vi "Constants.vi"() -> ()   [LabVIEW 2020, in "Ballard MIL-STD-1553 Scripting.lvlib"]
doc: "Use this Global VI to access the GUIDs assigned to the page resources of the Custom Device."
uses:
  Ballard MIL-STD-1553 Scripting.lvlib
panel:
  in  "Tab Control":enum32{"GUIDs", "Constants", "Properties"}(tab)
  in  "GUID.Error Count Channel":string="28D1D890-3AED-4F6D-A978-AD9A95C11628"
  in  "GUID.Status Section":string="1E0B5C0B-62AA-4583-9D0D-4E49A372EA3D"
  in  "GUID.Command Channel":string="F3C769CE-2055-47DC-98AC-89CDFED404B4"
  in  "GUID.Acyclic Frames":string="E577908A-4C92-429B-8C68-9740E425B266"
  in  "GUID.Timestamp Channel":string="4F0EA705-FD0A-4F01-AD6C-880781D6ED5B"
  in  "GUID.Status Word":string="7948DA20-805D-45D0-914D-274A69BA1942"
  in  "GUID.Trigger Channel":string="9F1749FA-E57B-4A2B-A4F8-443BB28943E1"
  in  "GUID.Message":string="2151C088-5813-42CA-818D-390AC9DDD1E2"
  in  "GUID.Subaddress":string="7E2EB233-E0C6-4644-BE22-C64B35DA4442"
  in  "GUID.Remote Terminal":string="D816BAC3-B801-4086-8FF2-44DEB0EE8E0A"
  in  "GUID.Bus Controller":string="B770364E-A524-47A4-BD2C-84D1536BF350"
  in  "GUID.Configuration Files":string="7D28FA5F-1BE9-42BA-9030-384369A394FD"
  in  "GUID.Channel":string="99523C72-475C-4B9B-9BFE-43F700A8EEC0"
  in  "GUID.Port":string="E61AF0D3-0C83-483A-A06B-B537FBE76C23"
  in  "GUID.Custom Device":string="96479D8D-68C1-4D19-959D-E0FE38040076"
  in  "Word Error Count":string="Word Error Count"
  in  "Monitor Error Count":string="Monitor Error Count"
  in  "Parity Error Count":string="Parity Error Count"
  in  "Manchester Error Count":string="Manchester Error Count"
  in  "Improper Number of Words Error Count":string="Improper Number of Words Error Count"
  in  "Wrong Sync Error Count":string="Wrong Sync Error Count"
  in  "General Protocol Error Count":string="General Protocol Error Count"
  in  "Unconfigured Frames Count":string="Unconfigured Frames Count"
  in  "PXI Slot Number":string="PXI Slot Number"
  in  "Card Number":string="Card Number"
  in  "Acyclic Frames":string="Acyclic Frames"
  in  "Timestamp":string="Timestamp"
  in  "Trigger":string="Trigger"
  in  "Status":string="Status"
  in  "Remote Terminal":string="Remote Terminal"
  in  "Stop":string="Stop"
  in  "Start":string="Start"
  in  "Bus Controller":string="Bus Controller"
  in  "Configuration Files":string="Configuration Files"
  in  "Channel":string="Channel"
  in  "Port":string="Port"
  in  "Prop.Mode.Code":string="modeCode"
  in  "Prop.Message.Type":string="messageType"
  in  "Prop.Direction":string="direction"
  in  "Prop.Acyclic.Frame.Name":string="acyclicFrameName"
  in  "Prop.Message.Name":string="messageName"
  in  "Prop.Number.Of.Words":string="numberOfWords"
  in  "Prop.Parameter":string="parameter"
  in  "Prop.Unit":string="unit"
  in  "Prop.Offset":string="offset"
  in  "Prop.Scale":string="scale"
  in  "Prop.Signed":string="signed"
  in  "Prop.Encoding":string="encoding"
  in  "Prop.SizeInBits":string="numberOfBits"
  in  "Prop.StartIndex":string="startBit"
  in  "Prop.DefaultValue":string="defaultValue"
  in  "Prop.Name":string="name"
  in  "Prop.Subaddress":string="subAddress"
  in  "Prop.Terminal.Address":string="terminalAddress"
  in  "Prop.Parameters.File":string="Win Parameters File Path"
  in  "Prop.Hardware.Configuration.File":string="Hardware Configuration File"
  in  "Prop.PXI.Slot.Number":string="PXI Slot Number"
  in  "Prop.Initialization.Method":string="Initialization Method"
  in  "Prop.Core.Number":string="core number"
  in  "Prop.Card.Number":string="card number"
  in  "Compiled.Settings":string="Compiled.Settings"
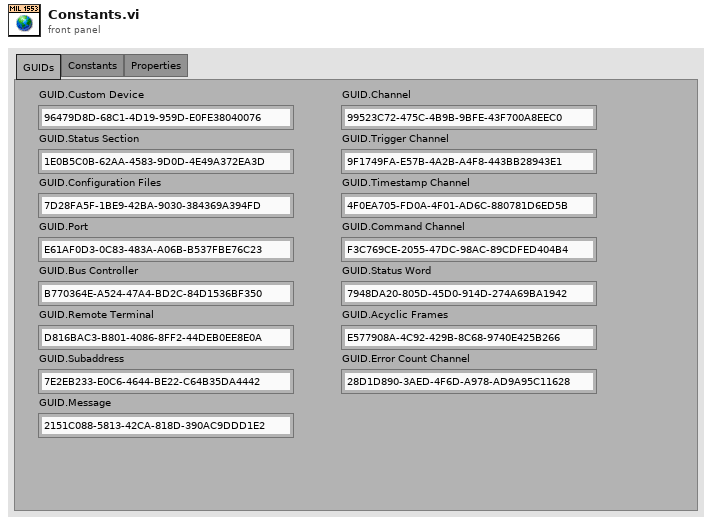
[diagram p1: front panel]
diagram:
